vi "Write config to front panel.vi"(3 "error in (no error)":errorcluster, 4 "frames in":u8[][](array[numeric]), 5 "FP ref in":T1) -> (0 "error out":errorcluster)   [LabVIEW 2020]
uses:
  Typedefs/Front Panel Object References.ctl
  Typedefs/LED mode.ctl
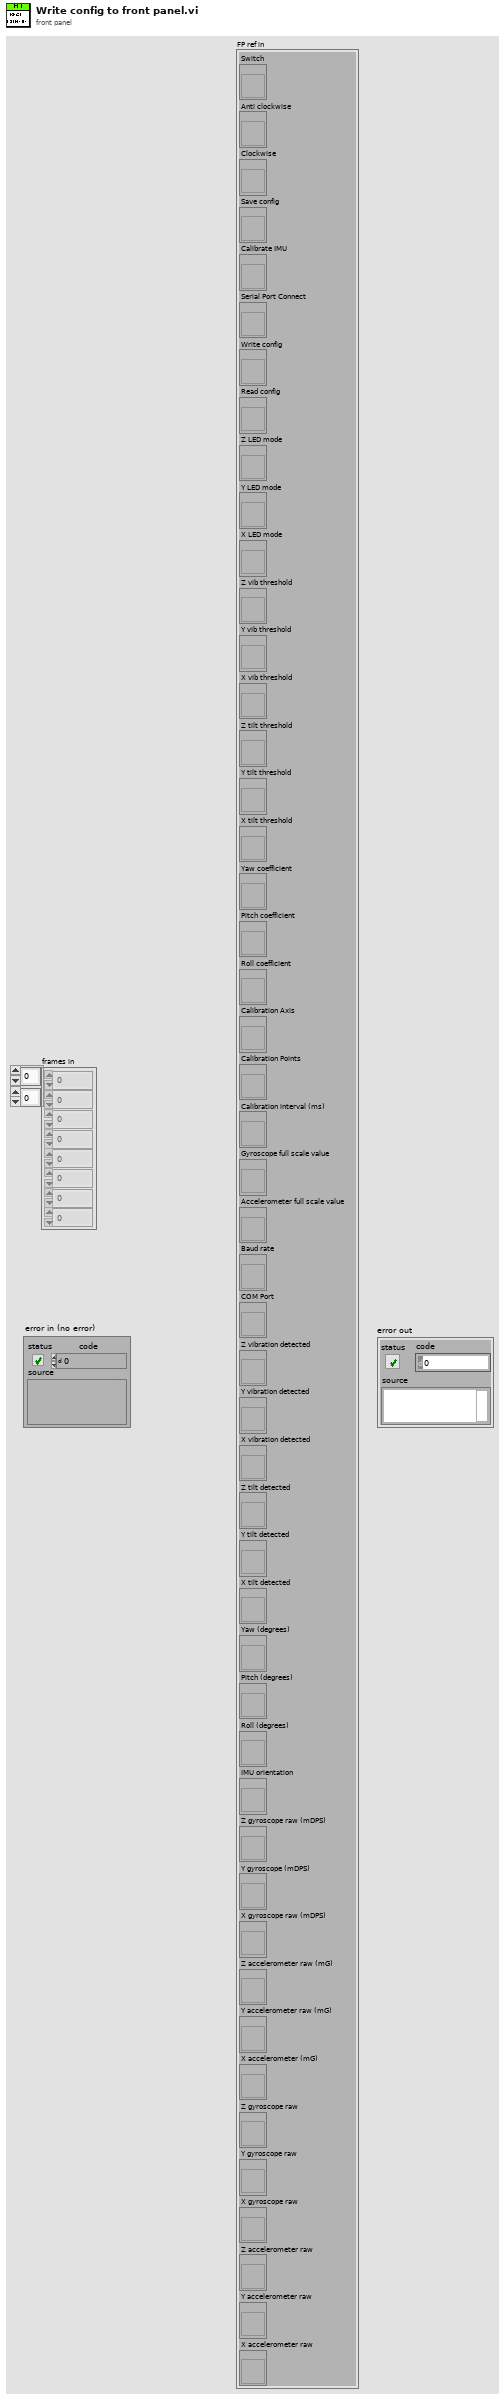
[diagram p1: front panel]
types:
  T1 = typedef "Front Panel Object References.ctl" = cluster{"Switch":refnum<vi>, "Anti clockwise":refnum<vi>, "Clockwise":refnum<vi>, "Save config":refnum<vi>, "Calibrate IMU":refnum<vi>, "Serial Port Connect":refnum<vi>, "Write config":refnum<vi>, "Read config":refnum<vi>, "Z LED mode":refnum<vi>, "Y LED mode":refnum<vi>, "X LED mode":refnum<vi>, "Z vib threshold":refnum<vi>, "Y vib threshold":refnum<vi>, "X vib threshold":refnum<vi>, "Z tilt threshold":refnum<vi>, "Y tilt threshold":refnum<vi>, "X tilt threshold":refnum<vi>, "Yaw coefficient":refnum<vi>, "Pitch coefficient":refnum<vi>, "Roll coefficient":refnum<vi>, "Calibration Axis":refnum<vi>, "Calibration Points":refnum<vi>, "Calibration interval (ms)":refnum<vi>, "Gyroscope full scale value":refnum<vi>, "Accelerometer full scale value":refnum<vi>, "Baud rate":refnum<vi>, "COM Port":refnum<vi>, "Z vibration detected":refnum<vi>, "Y vibration detected":refnum<vi>, "X vibration detected":refnum<vi>, "Z tilt detected":refnum<vi>, "Y tilt detected":refnum<vi>, "X tilt detected":refnum<vi>, "Yaw (degrees)":refnum<vi>, "Pitch (degrees)":refnum<vi>, "Roll (degrees)":refnum<vi>, "IMU orientation":refnum<vi>, "Z gyroscope raw (mDPS)":refnum<vi>, "Y gyroscope (mDPS)":refnum<vi>, "X gyroscope raw (mDPS)":refnum<vi>, "Z accelerometer raw (mG)":refnum<vi>, "Y accelerometer raw (mG)":refnum<vi>, "X accelerometer (mG)":refnum<vi>, "Z gyroscope raw":refnum<vi>, "Y gyroscope raw":refnum<vi>, "X gyroscope raw":refnum<vi>, "Z accelerometer raw":refnum<vi>, "Y accelerometer raw":refnum<vi>, "X accelerometer raw":refnum<vi>}
  T2 = enum16{"250DPS", "500DPS", "1000DPS", "2000DPS"}[]
  T3 = enum16{"X positive", "X neagtive", "Y positive", "Y negative", "Z positive", "Z negative"}[]
  T4 = enum16{"X positive", "X neagtive", "Y positive", "Y negative", "Z positive", "Z negative"}
  T5 = typedef "LED mode.ctl" = enum16{"Tilt detection", "Vibration detection", "Accelerometer magnitude", "Gyroscope magnitude", "GPIO test", "PWM test"}
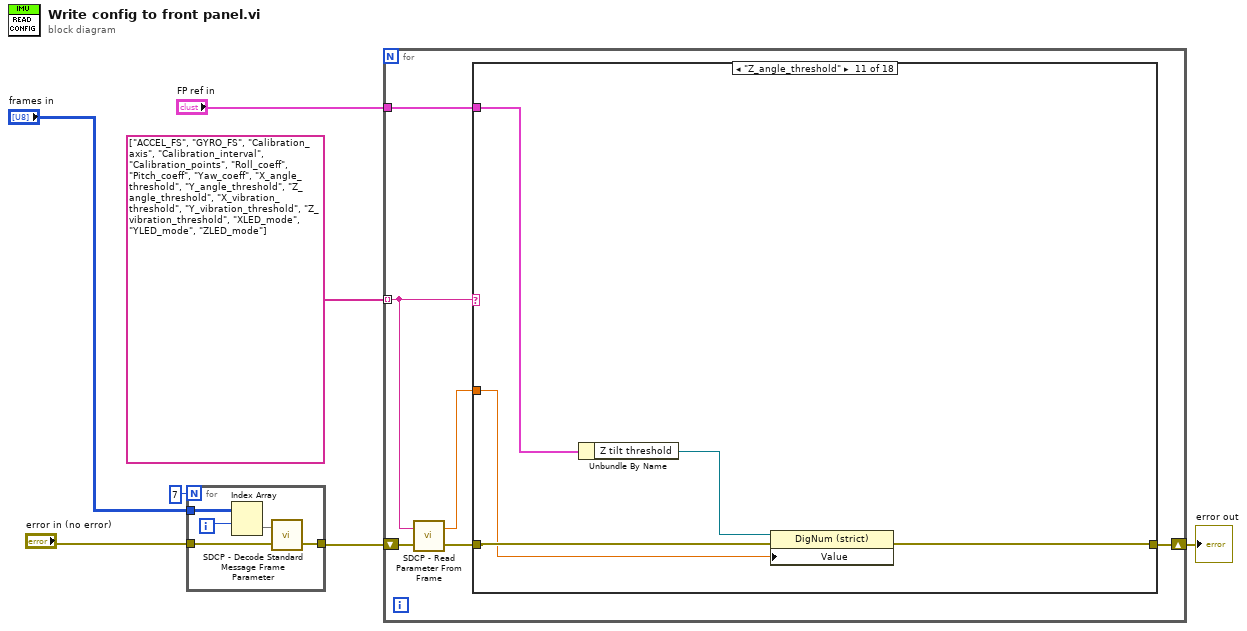
[diagram p0: block diagram]
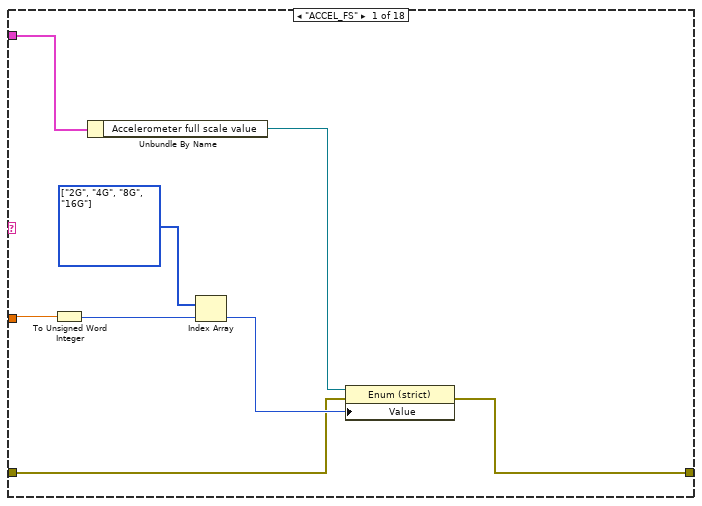
[diagram p2: hidden frame]
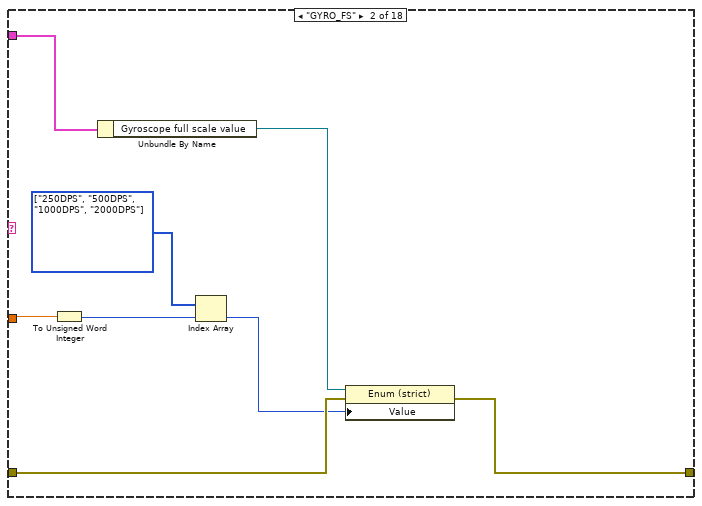
[diagram p3: hidden frame]
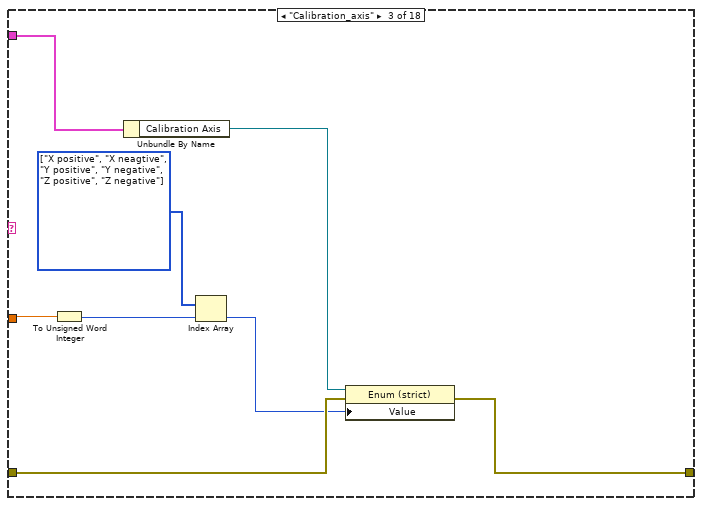
[diagram p4: hidden frame]
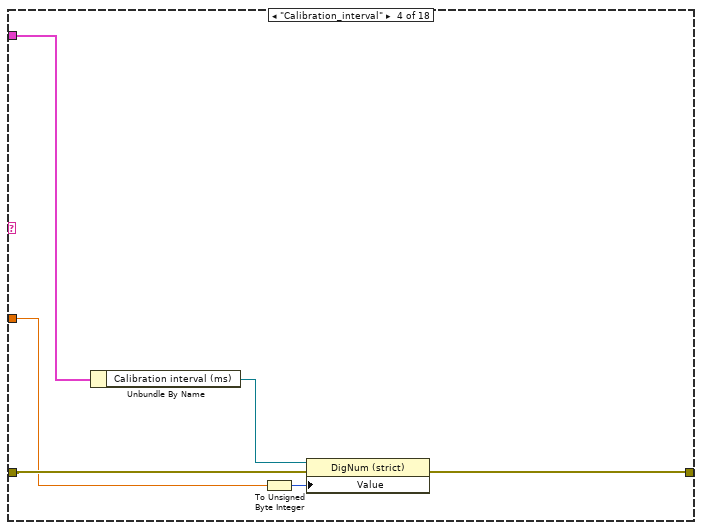
[diagram p5: hidden frame]
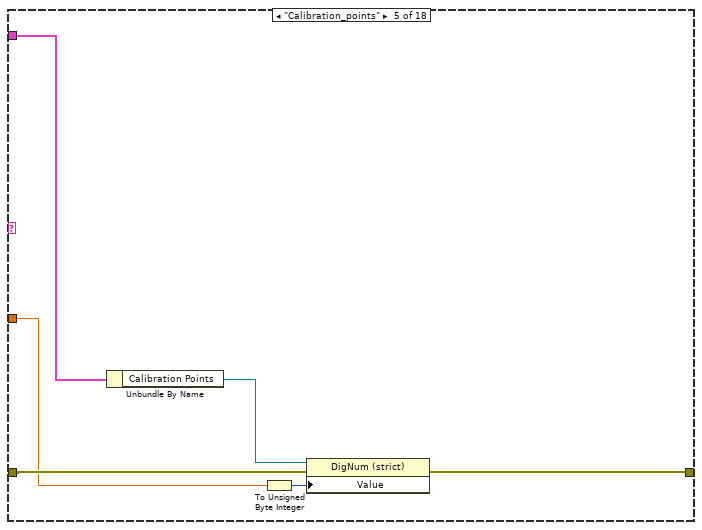
[diagram p6: hidden frame]
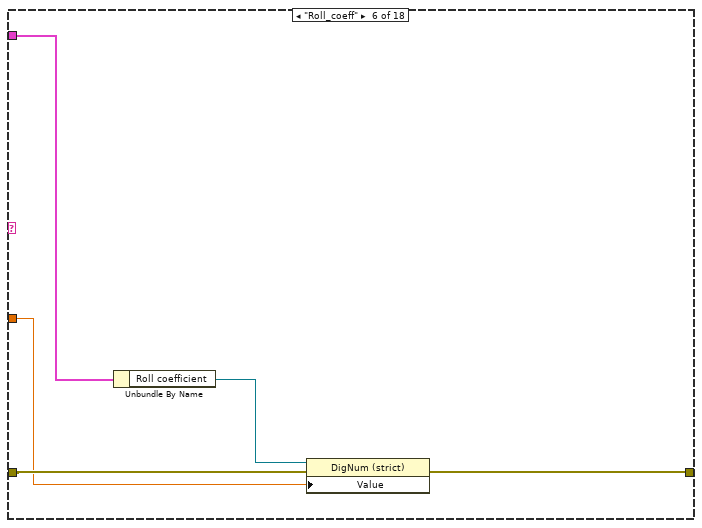
[diagram p7: hidden frame]
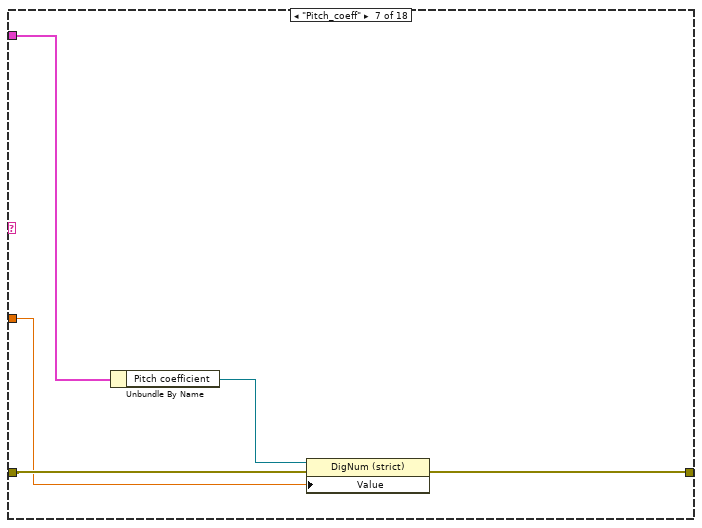
[diagram p8: hidden frame]
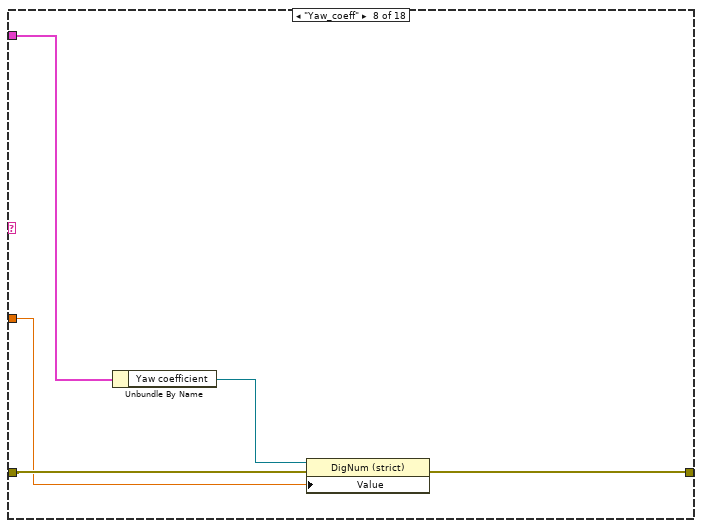
[diagram p9: hidden frame]
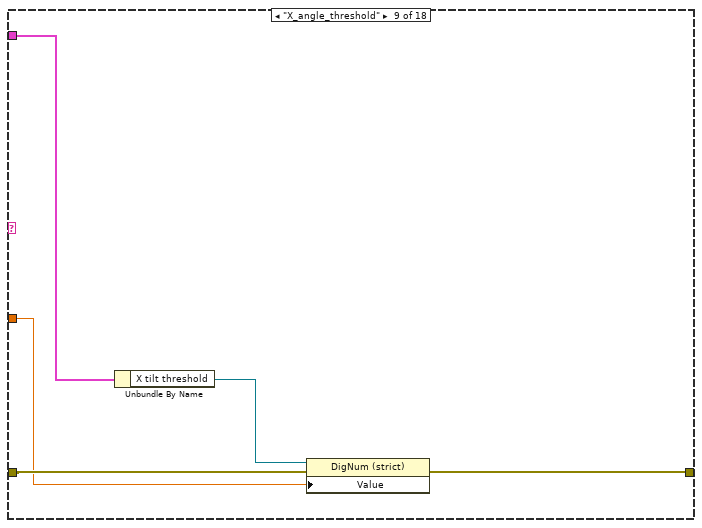
[diagram p10: hidden frame]
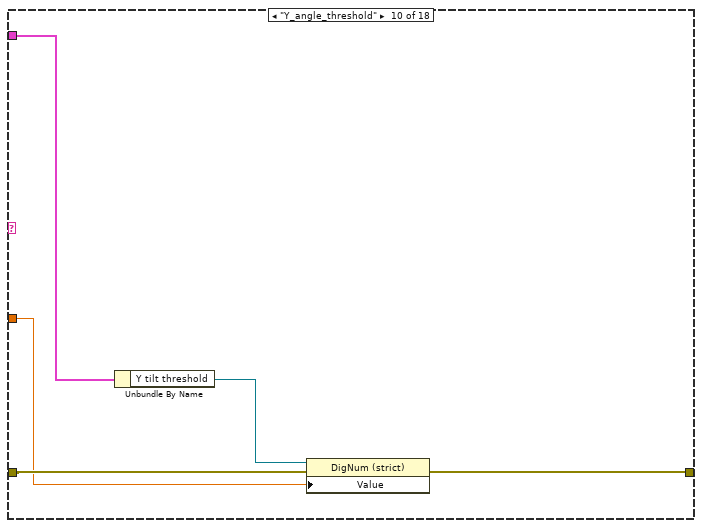
[diagram p11: hidden frame]
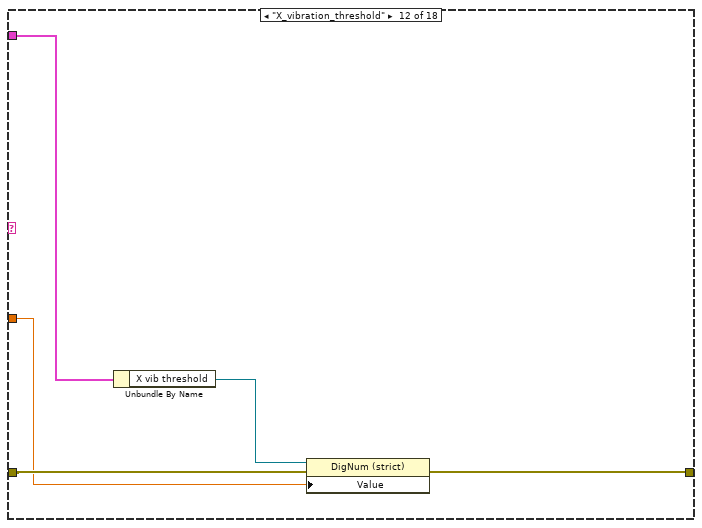
[diagram p12: hidden frame]
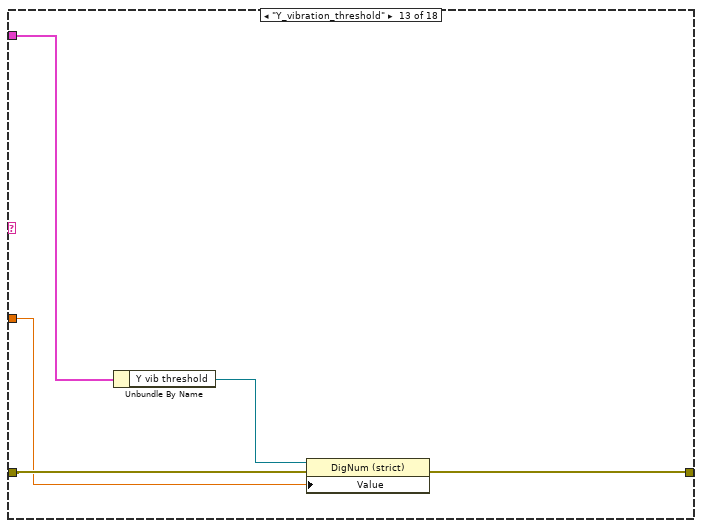
[diagram p13: hidden frame]
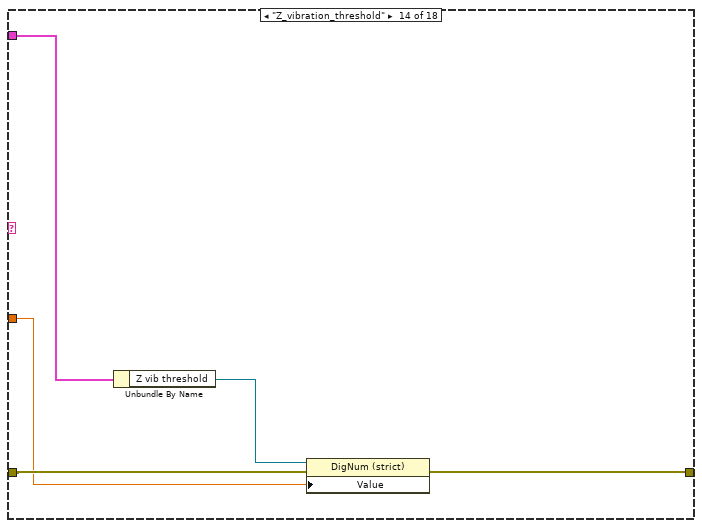
[diagram p14: hidden frame]
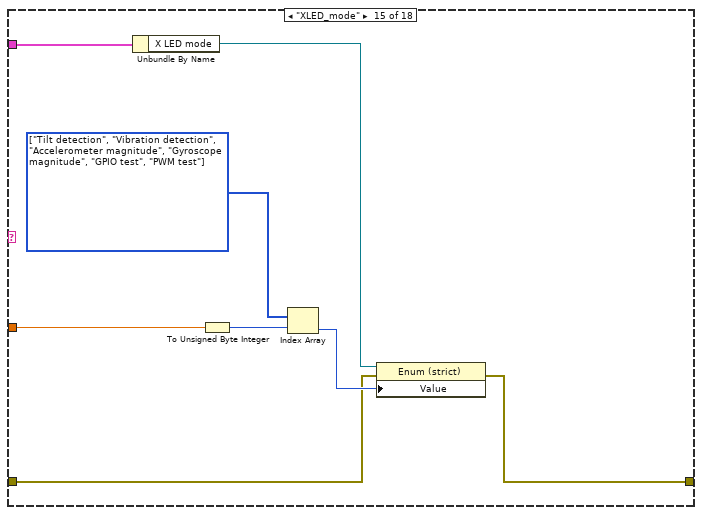
[diagram p15: hidden frame]
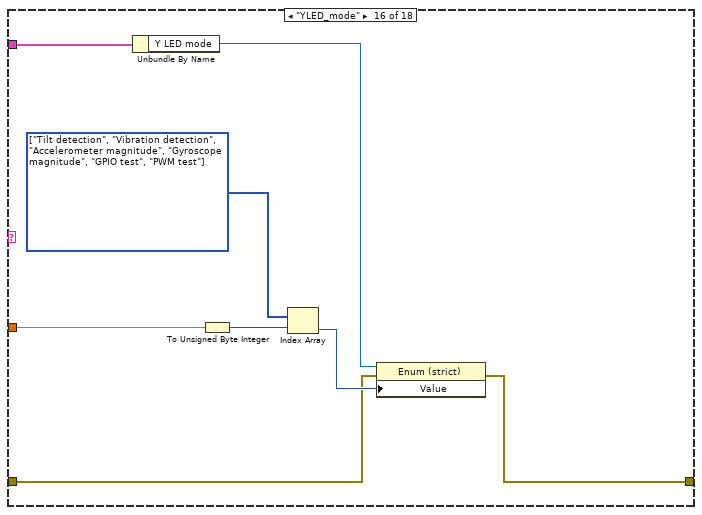
[diagram p16: hidden frame]
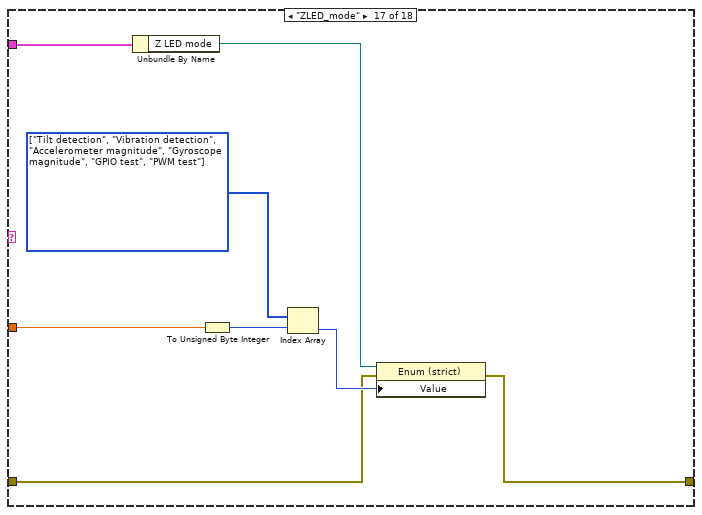
[diagram p17: hidden frame]
diagram:
  n1 = for {
    N: 7 -> [_]
    tunnel: "frames in" -> [w12]
    tunnel: "error in (no error)" -> [w10]
    tunnel: [w8] -> w4
    i -> [w9]
    n2 = Index Array(array=w12, index (row)=w9) -> (element=w11:u8[])  [unwired: 1 in]
    n3 = call "SDCP - Decode Standard Message Frame Parameter.vi"("error in (no error)"=w10, "Bytes in"=w11) -> ("error out"=w8:errorcluster)  [unwired: 1 out]
  }
  n4 = for {
    tunnel: string[] ["ACCEL_FS", "GYRO_FS", "Calibration_axis", "Calibration_interval", "Calibration_points", "Roll_coeff", "Pitch_coeff", "Yaw_coeff", "X_angle_threshold", "Y_angle_threshold", "Z_angle_threshold", "X_vibration_threshold", "Y_vibration_threshold", "Z_vibration_threshold", "XLED_mode", "YLED_mode", "ZLED_mode"] -> [w16] mode=indexing
    shift-right: [w14] -> w1
    shift-left: w4 -> [w18]
    tunnel: "FP ref in" -> [w13]
    n5 = call "SDCP - Read Parameter From Frame.vi"("error in (no error)"=w18, "Parameter"=w16) -> ("error out"=w17:errorcluster, "Value"=w15:dbl)
    n6 = case shown="\"Z_angle_threshold\"" w16 {
      tunnel: w17 -> [w20 w30 w38 w46 w52 w57 w62 w67 w72 w77 w82 w87 w92 w97 w101 w109 w117 w124]
      tunnel: w15 -> [w26 w34 w42 w44 w50 w55 w60 w65 w70 w75 w80 w85 w90 w95 w104 w112 w120 _]
      tunnel: [w19 w29 w37 w43 w49 w56 w61 w66 w71 w76 w81 w86 w91 w96 w100 w108 w116 w124] -> w14
      tunnel: w13 -> [w25 w33 w41 w48 w54 w59 w64 w69 w74 w79 w84 w89 w94 w99 w107 w115 w123 _]
      frame "ACCEL_FS" {
        w22 = enum16{"2G", "4G", "8G", "16G"}[] [enum."2G", enum."4G", enum."8G", enum."16G"] items=["2G", "4G", "8G", "16G"]
        n7 = To Unsigned Word Integer(number=w26) -> (unsigned 16bit integer=w23:u16)
        n8 = Unbundle By Name(w25) -> ("Accelerometer full scale value"=w24:refnum<vi>)
        n9 = Index Array(array=w22, index=w23) -> (element=w21:enum16{"2G", "4G", "8G", "16G"})
        n10 = property class="Enum (strict)"(reference=w24, error in=w20, "Value"=w21) -> (error out=w19:errorcluster)  [unwired: 1 out]
      }
      frame "GYRO_FS" {
        w28 = T2 [enum."250DPS", enum."500DPS", enum."1000DPS", enum."2000DPS"] items=["250DPS", "500DPS", "1000DPS", "2000DPS"]
        n11 = To Unsigned Word Integer(number=w34) -> (unsigned 16bit integer=w31:u16)
        n12 = Unbundle By Name(w33) -> ("Gyroscope full scale value"=w32:refnum<vi>)
        n13 = Index Array(array=w28, index=w31) -> (element=w27:enum16{"250DPS", "500DPS", "1000DPS", "2000DPS"})
        n14 = property class="Enum (strict)"(reference=w32, error in=w30, "Value"=w27) -> (error out=w29:errorcluster)  [unwired: 1 out]
      }
      frame "Calibration_axis" {
        w36 = T3 [enum."X positive", enum."X neagtive", enum."Y positive", enum."Y negative", enum."Z positive", enum."Z negative"] items=["X positive", "X neagtive", "Y positive", "Y negative", "Z positive", "Z negative"]
        n15 = To Unsigned Word Integer(number=w42) -> (unsigned 16bit integer=w39:u16)
        n16 = Unbundle By Name(w41) -> ("Calibration Axis"=w40:refnum<vi>)
        n17 = Index Array(array=w36, index=w39) -> (element=w35:T4)
        n18 = property class="Enum (strict)"(reference=w40, error in=w38, "Value"=w35) -> (error out=w37:errorcluster)  [unwired: 1 out]
      }
      frame "Calibration_interval" {
        n19 = Unbundle By Name(w48) -> ("Calibration interval (ms)"=w47:refnum<vi>)
        n20 = To Unsigned Byte Integer(number=w44) -> (unsigned 8bit integer=w45:u8)
        n21 = property class="DigNum (strict)"(reference=w47, error in=w46, "Value"=w45) -> (error out=w43:errorcluster)  [unwired: 1 out]
      }
      frame "Calibration_points" {
        n22 = Unbundle By Name(w54) -> ("Calibration Points"=w53:refnum<vi>)
        n23 = To Unsigned Byte Integer(number=w50) -> (unsigned 8bit integer=w51:u8)
        n24 = property class="DigNum (strict)"(reference=w53, error in=w52, "Value"=w51) -> (error out=w49:errorcluster)  [unwired: 1 out]
      }
      frame "Roll_coeff" {
        n25 = Unbundle By Name(w59) -> ("Roll coefficient"=w58:refnum<vi>)
        n26 = property class="DigNum (strict)"(reference=w58, error in=w57, "Value"=w55) -> (error out=w56:errorcluster)  [unwired: 1 out]
      }
      frame "Pitch_coeff" {
        n27 = Unbundle By Name(w64) -> ("Pitch coefficient"=w63:refnum<vi>)
        n28 = property class="DigNum (strict)"(reference=w63, error in=w62, "Value"=w60) -> (error out=w61:errorcluster)  [unwired: 1 out]
      }
      frame "Yaw_coeff" {
        n29 = Unbundle By Name(w69) -> ("Yaw coefficient"=w68:refnum<vi>)
        n30 = property class="DigNum (strict)"(reference=w68, error in=w67, "Value"=w65) -> (error out=w66:errorcluster)  [unwired: 1 out]
      }
      frame "X_angle_threshold" {
        n31 = Unbundle By Name(w74) -> ("X tilt threshold"=w73:refnum<vi>)
        n32 = property class="DigNum (strict)"(reference=w73, error in=w72, "Value"=w70) -> (error out=w71:errorcluster)  [unwired: 1 out]
      }
      frame "Y_angle_threshold" {
        n33 = Unbundle By Name(w79) -> ("Y tilt threshold"=w78:refnum<vi>)
        n34 = property class="DigNum (strict)"(reference=w78, error in=w77, "Value"=w75) -> (error out=w76:errorcluster)  [unwired: 1 out]
      }
      frame "Z_angle_threshold" {
        n35 = Unbundle By Name(w84) -> ("Z tilt threshold"=w83:refnum<vi>)
        n36 = property class="DigNum (strict)"(reference=w83, error in=w82, "Value"=w80) -> (error out=w81:errorcluster)  [unwired: 1 out]
      }
      frame "X_vibration_threshold" {
        n37 = Unbundle By Name(w89) -> ("X vib threshold"=w88:refnum<vi>)
        n38 = property class="DigNum (strict)"(reference=w88, error in=w87, "Value"=w85) -> (error out=w86:errorcluster)  [unwired: 1 out]
      }
      frame "Y_vibration_threshold" {
        n39 = Unbundle By Name(w94) -> ("Y vib threshold"=w93:refnum<vi>)
        n40 = property class="DigNum (strict)"(reference=w93, error in=w92, "Value"=w90) -> (error out=w91:errorcluster)  [unwired: 1 out]
      }
      frame "Z_vibration_threshold" {
        n41 = Unbundle By Name(w99) -> ("Z vib threshold"=w98:refnum<vi>)
        n42 = property class="DigNum (strict)"(reference=w98, error in=w97, "Value"=w95) -> (error out=w96:errorcluster)  [unwired: 1 out]
      }
      frame "XLED_mode" {
        w105 = T5[] [enum."Tilt detection", enum."Vibration detection", enum."Accelerometer magnitude", enum."Gyroscope magnitude", enum."GPIO test", enum."PWM test"] items=["Tilt detection", "Vibration detection", "Accelerometer magnitude", "Gyroscope magnitude", "GPIO test", "PWM test"]
        n43 = Unbundle By Name(w107) -> ("X LED mode"=w106:refnum<vi>)
        n44 = To Unsigned Byte Integer(number=w104) -> (unsigned 8bit integer=w103:u8)
        n45 = Index Array(array=w105, index=w103) -> (element=w102:T5)
        n46 = property class="Enum (strict)"(reference=w106, error in=w101, "Value"=w102) -> (error out=w100:errorcluster)  [unwired: 1 out]
      }
      frame "YLED_mode" {
        w113 = T5[] [enum."Tilt detection", enum."Vibration detection", enum."Accelerometer magnitude", enum."Gyroscope magnitude", enum."GPIO test", enum."PWM test"] items=["Tilt detection", "Vibration detection", "Accelerometer magnitude", "Gyroscope magnitude", "GPIO test", "PWM test"]
        n47 = Unbundle By Name(w115) -> ("Y LED mode"=w114:refnum<vi>)
        n48 = To Unsigned Byte Integer(number=w112) -> (unsigned 8bit integer=w111:u8)
        n49 = Index Array(array=w113, index=w111) -> (element=w110:T5)
        n50 = property class="Enum (strict)"(reference=w114, error in=w109, "Value"=w110) -> (error out=w108:errorcluster)  [unwired: 1 out]
      }
      frame "ZLED_mode" {
        w121 = T5[] [enum."Tilt detection", enum."Vibration detection", enum."Accelerometer magnitude", enum."Gyroscope magnitude", enum."GPIO test", enum."PWM test"] items=["Tilt detection", "Vibration detection", "Accelerometer magnitude", "Gyroscope magnitude", "GPIO test", "PWM test"]
        n51 = Unbundle By Name(w123) -> ("Z LED mode"=w122:refnum<vi>)
        n52 = To Unsigned Byte Integer(number=w120) -> (unsigned 8bit integer=w119:u8)
        n53 = Index Array(array=w121, index=w119) -> (element=w118:T5)
        n54 = property class="Enum (strict)"(reference=w122, error in=w117, "Value"=w118) -> (error out=w116:errorcluster)  [unwired: 1 out]
      }
      frame Default {
      }
    }
  }
  "error out" <- w1
